vi "Get Index Directory Path.vi"(8 "error in (no error)":errorcluster) -> (0 "error out":errorcluster, 3 "Index Directory":path)   [LabVIEW 2020, in "Utilities.lvlib"]
doc: "Generates the default configuration path. \nWhen called from the development environement, the default config path is the /Config relative to the project path.\nWhen called from a built exe the default config path is at C:\\Users\\<username>\\AppData\\Local\\<CompanyName>\\<ProductName> where company name and product name are the ones configured in the build specification.\nOn Linux the default config directory is \\home\\lvuser\\natinst\\bin\\config."
uses:
  Utilities.lvlib
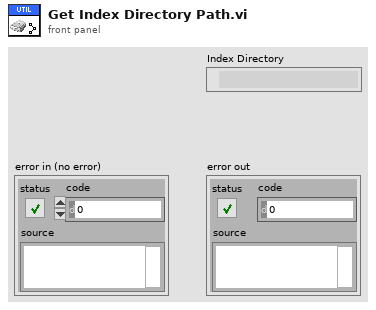
[diagram p1: front panel]
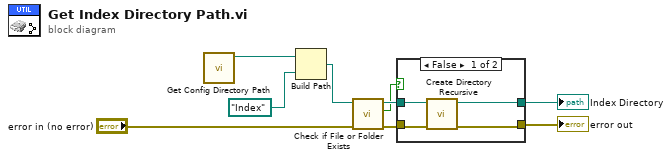
[diagram p0: block diagram]
diagram:
  n1 = call "Get Config Directory Path.vi"() -> ("appended path"=w3:path)  [unwired: 11 in]
  n2 = Build Path(base path=w3, name or relative path=path "Index") -> (appended path=w2:path)
  n3 = call <vilib>:"Check if File or Folder Exists.vi"("error in (no error)"="error in (no error)", "path"=w2) -> ("error out"=w5:errorcluster, "file or folder exists?"=w4:bool, "dup path"=w6:path)  [unwired: 7 in]
  n4 = case shown="False" w4 {
    tunnel: [w11 w14] -> w9
    tunnel: [w10 w15] -> w7
    tunnel: w6 -> [w13 w15]
    tunnel: w5 -> [w12 w14]
    frame False {
      n5 = call <vilib>:"Create Directory Recursive.vi"("error in (no error)"=w12, "directory"=w13) -> ("error out"=w11:errorcluster, "directory copy"=w10:path)  [unwired: 3 in, 1 out]
    }
    frame True {
    }
  }
  "Index Directory" <- w7
  "error out" <- w9
